vi "Helpers.vi"() -> ()   [LabVIEW 2018, in "Main.lvlib"]
uses:
  Main.lvlib
panel:
  in  "VI Launch":string="VI to launch:\n%s"
  in  "Edited":string="*Restart required to reload*"
  in  "No Items":string="<No Applications Setup>"
  in  "No Apps":string="Press \"Configure\" to edit.\n\n*Restart required to reload*"
  in  "No path":string="[app] path key missing.\n%s\n*Restart required to reload*"
  in  "No VI":string="Unable to resolve VI path:\n%s\n*Restart required to reload*"
  in  "No Ini":string="File not found:\n%s\n*Restart required to reload*"
  in  "Startup Text":string="[apps]\n;- Applications to load, each key is a separated app.\n;- APP_NAME = CONFIG_PATH\n;-   APP_NAME:    Name of the application.\n;-   CONFIG_PATH: Path to configuration file (*.ini),\n;-                can be absolute or relative path and\n;-                must be a unique file for each app.\n\nDEMO = .\\Startup.ini\n\n;- Each CONFIG_PATH must be a unique settings file that\n;- contain an \"[app]\" section with a \"vi\" key to the\n;- qualified VI name to launch in either a\n;- Packed Project Library (*.lvlibp:*.vi) or\n;- Project Library (*.lvlib:*.vi)\n;-   [app]\n;-   ; vi = QUALIFIED_VI_NAME\n;-   vi = Demo.lvlibp:Module.vi    // Packed Library (Built)\n;-   vi = Demo.lvlib:Module.vi     // Project Library (Source)\n;- The VI path is resolved by searching the sub-directories\n;- of this Startup.ini path, first in '.\\Builds', then\n;- '.\\Modules' and finally the root dir '.\\' to locate the VI.\n;- The following is used for demo purposes only.\n\n[app]\nvi = Demo.lvlib:Demo.vi\n; vi = Demo.lvlibp:Demo.vi"
  in  "No Startup":string="Startup.ini not found.\n\n--- Expected Path ---\n\n%s\n\n--- Example: Startup.ini ---\n[apps]\n; APP_NAME = CONFIG_PATH\nAPP1 = .\\\\Configs\\\\App.ini"
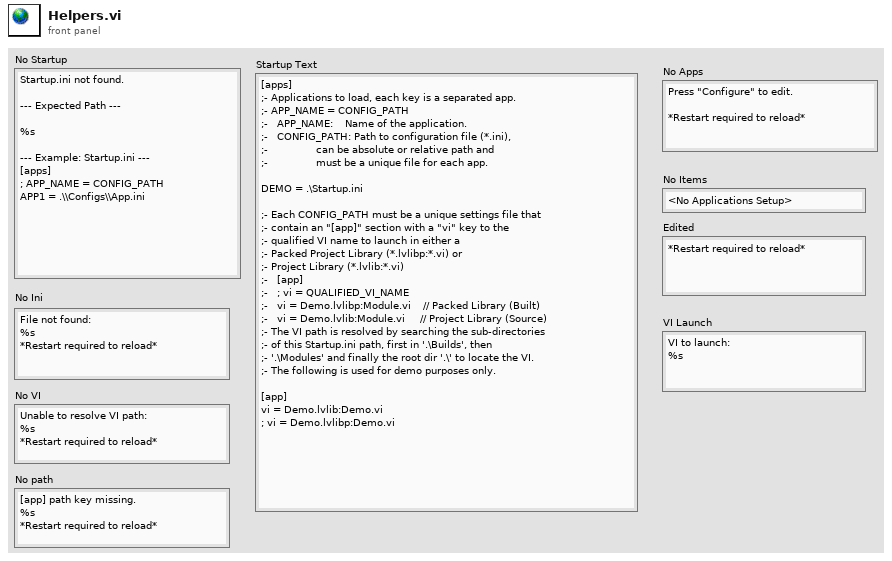
[diagram p1: front panel]
diagram:
